vi "unregUserEvent.vi"(8 "error in (no error)":errorcluster, 11 "tcpServerCmd in":refnum<class "TcpServerCmd.lvclass">) -> (0 "error out":errorcluster, 3 "tcpServerCmd out":refnum<class "TcpServerCmd.lvclass">)   [LabVIEW 2018, in "TcpServerCmd.lvclass"]
doc: "Unregister User Events."
uses:
  TcpServerCmd.lvclass
  TcpServerCmd.lvclass/TcpServerCmd.ctl
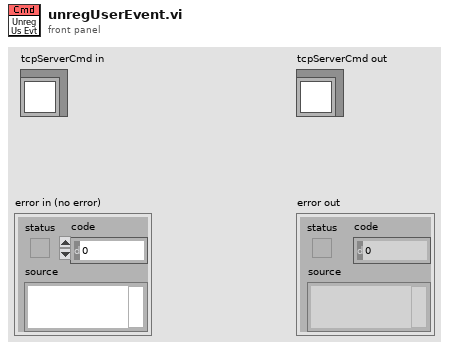
[diagram p1: front panel]
types:
  T1 = typedef "TcpServerCmd.lvclass/userEventTypeDef.ctl" = cluster{"CmdRead":refnum<user-event>, "CmdWrite":refnum<user-event>, "EvtRead":refnum<user-event>, "EvtWrite":refnum<user-event>, "GenRead":refnum<user-event>, "GenWrite":refnum<user-event>}
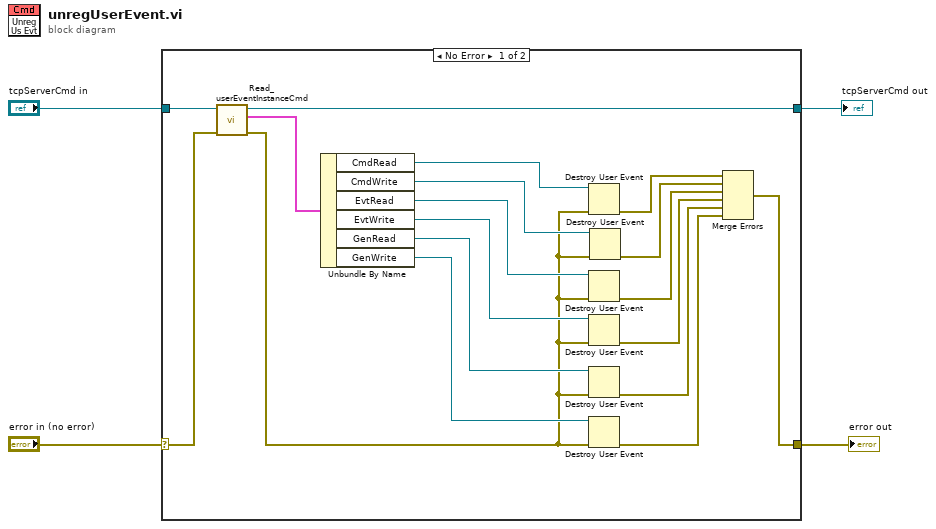
[diagram p0: block diagram]
diagram:
  n1 = case shown="No Error" "error in (no error)" {
    selector: "error in (no error)" -> [w20 w24]
    tunnel: [w18 w24] -> w3
    tunnel: [w21 w23] -> w1
    tunnel: "tcpServerCmd in" -> [w22 w23]
    frame No Error {
      n2 = call "Read_userEventInstanceCmd.vi"("error in (no error)"=w20, "TcpServerCmd in"=w22) -> ("error out"=w5:errorcluster, "userEventInstance"=w19:T1, "TcpServerCmd out"=w21:refnum<class "TcpServerCmd.lvclass">)  [unwired: 7 in]
      n3 = Unbundle By Name(w19) -> ("CmdRead"=w16:refnum<user-event>, "CmdWrite"=w15:refnum<user-event>, "EvtRead"=w14:refnum<user-event>, "EvtWrite"=w12:refnum<user-event>, "GenRead"=w11:refnum<user-event>, "GenWrite"=w10:refnum<user-event>)
      n4 = Destroy User Event(user event=w16, error in=w5) -> (error out=w17:errorcluster)
      n5 = Destroy User Event(user event=w14, error in=w5) -> (error out=w9:errorcluster)
      n6 = Destroy User Event(user event=w12, error in=w5) -> (error out=w8:errorcluster)
      n7 = Destroy User Event(user event=w11, error in=w5) -> (error out=w7:errorcluster)
      n8 = Destroy User Event(user event=w10, error in=w5) -> (error out=w6:errorcluster)
      n9 = Destroy User Event(user event=w15, error in=w5) -> (error out=w13:errorcluster)
      n10 = Merge Errors(w17, w13, w9, w8, w7, w6) -> (w18:errorcluster)
    }
    frame Error {
    }
  }
  "error out" <- w3
  "tcpServerCmd out" <- w1
